vi "1.2.1-ParseYPR.vi"(9 "ASCII: VNYPR,":u8[](array[numeric])=[86, 78, 89, 80, 82, 44], 10 "Serial Byte":u8) -> (1 "Yaw":i16)   [LabVIEW 2010]
doc: "This VI parses Yaw, Pitch, and Roll (YPR) data from the VectorNav. In response to a YPR Read Request, the VectorNav will reply in the form \"$VNYPR,XX,-XXX.XX,-XXX.XX,+XXX.XX*XX\" (where X is a digit from 0-9). This string is in the form \"$<command type>,<access ID>, <yaw>,<pitch>,<roll>\".\n\nThe VI first waits for a $, then checks to make sure it has read \"VNYPR,\" correctly, then adds up each of the XX values and saves them appropriately. Since it receives these values one byte at a time , it must do some simple fixed point math to make sure the appropriate decimal value is saved."
uses:
  1.2.1-ParseYPR.ctl
panel:
  out "Heading (out)":T1 {"Yaw" format="%.19g"; "Pitch" format="%.19g"; "Roll" format="%.19g"}
  in  "Heading (in)":T1 {"Yaw" format="%.42g"; "Pitch" format="%.42g"; "Roll" format="%.42g"}
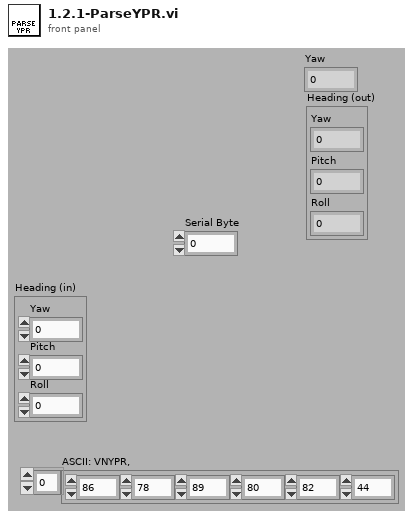
[diagram p1: front panel]
types:
  T1 = cluster{"Yaw":fxp<+/-,32,20>, "Pitch":fxp<+/-,32,20>, "Roll":fxp<+/-,32,20>}
  T2 = typedef "1.2.1-ParseYPR.ctl" = enum16{"Wait for $", "Check VNYPR", "Read numbers"}
  T3 = enum16{"Initialize", "Yaw", "Pitch", "Roll", "Done"}
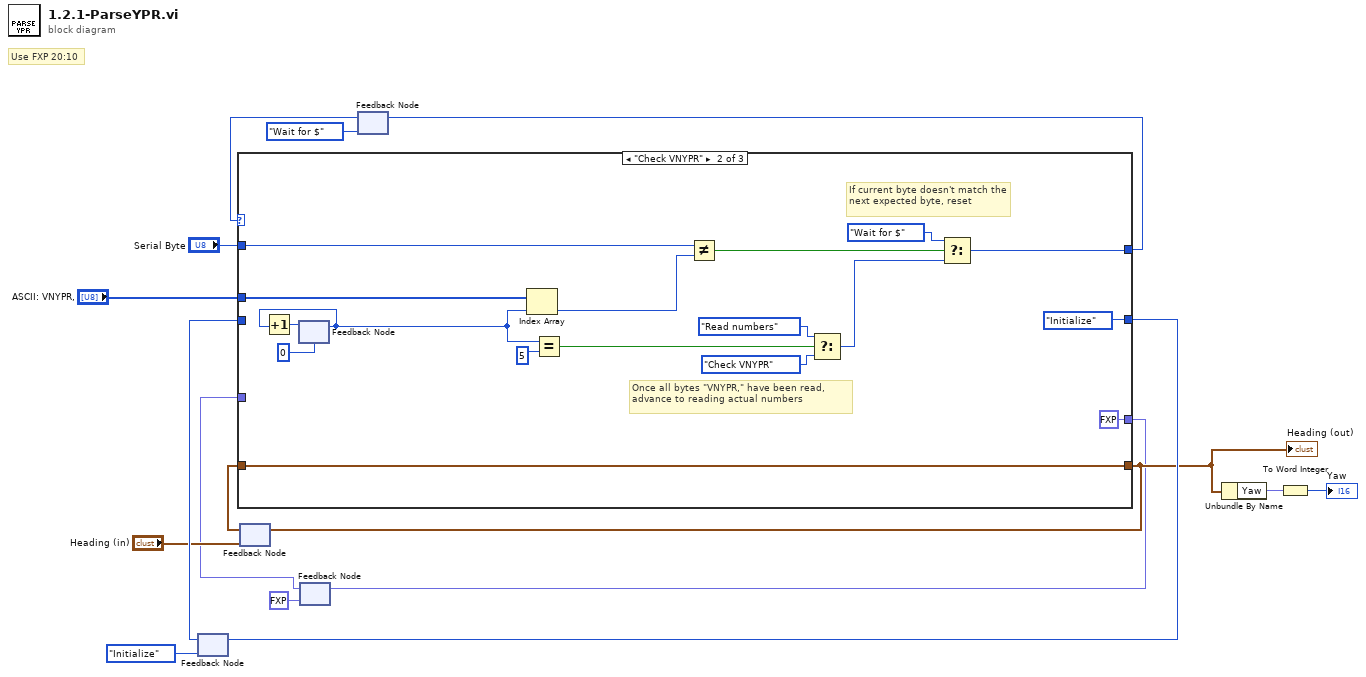
[diagram p0: block diagram]
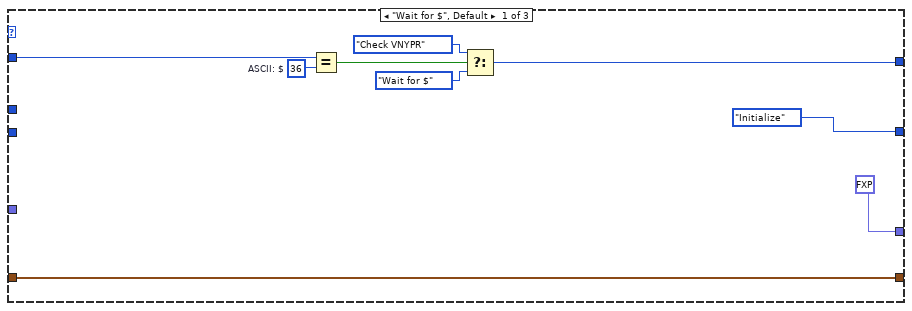
[diagram p2: hidden frame]
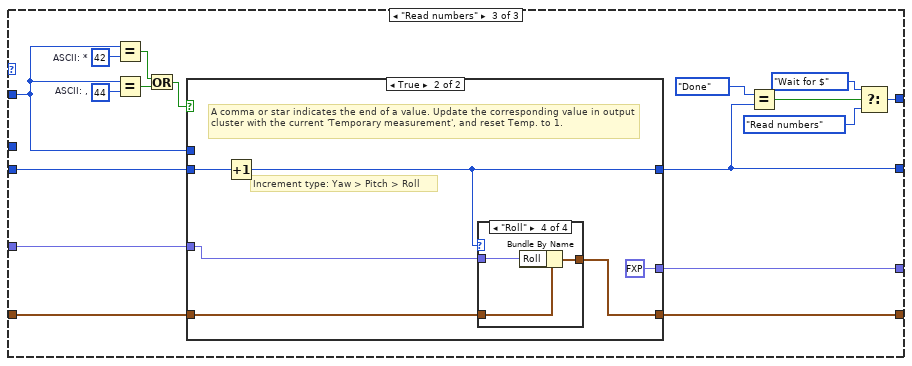
[diagram p3: hidden frame]
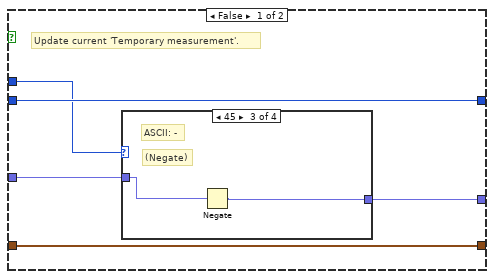
[diagram p4: hidden frame]
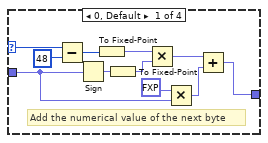
[diagram p5: hidden frame]
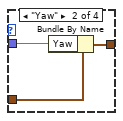
[diagram p9: hidden frame]
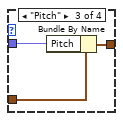
[diagram p10: hidden frame]
diagram:
  # "Use FXP 20:10"
  n1 = feedback #1(T3."Initialize" ("f")) -> (w11:T3)
  n2 = feedback #2("Heading (in)") -> (w5:T1)
  n3 = feedback #3(fxp<+/-,32,20> 1.0 ("Yaw")) -> (w3:fxp<+/-,32,20>)
  n4 = feedback #4(1.2.1-ParseYPR."Wait for $" ("1.3.1-ParseYPR")) -> (w14:T2)
  n5 = case shown="\"Check VNYPR\"" w14 {
    tunnel: [w22 w32 w47] -> w16
    tunnel: "Serial Byte" -> [w25 w39 w46]
    tunnel: [fxp<+/-,32,20> 1.0 ("Yaw") fxp<+/-,32,20> 1.0 ("Yaw") w48] -> w2
    tunnel: [w21 w40 w57] -> w4
    tunnel: w5 -> [w21 w40 w58]
    tunnel: [T3."Initialize" ("f") T3."Initialize" ("f") w55] -> w12
    tunnel: w11 -> [_ _ w56]
    tunnel: w3 -> [_ _ w43]
    tunnel: "ASCII: VNYPR," -> [_ w26 _]
    frame "Wait for $", Default {
      w24 = u8 36  # ASCII: $
      n6 = Equal?(x=w25, y=w24) -> (x = y?=w23:bool)
      n7 = Select(t=1.2.1-ParseYPR."Check VNYPR" ("1.3.1-ParseYPR"), s=w23, f=1.2.1-ParseYPR."Wait for $" ("1.3.1-ParseYPR")) -> (s? t:f=w22:T2)
    }
    frame "Check VNYPR" {
      # "If current byte doesn't match the next expected byte, reset"
      # "Once all bytes \"VNYPR,\" have been read, advance to reading actual numbers"
      n8 = feedback #5(0 ("Serial Byte")) -> (w27:i32)
      n9 = Increment(x=w27) -> (x+1=w28:i32)
      n10 = feedback-in #5(w28) -> ()
      n11 = Index Array(array=w26, index=w27) -> (element=w42:u8)
      n12 = Equal?(x=w27, y=5) -> (x = y?=w37:bool)
      n13 = Not Equal?(x=w39, y=w42) -> (x != y?=w41:bool)
      n14 = Select(t=1.2.1-ParseYPR."Read numbers" ("1.3.1-ParseYPR"), s=w37, f=1.2.1-ParseYPR."Check VNYPR" ("1.3.1-ParseYPR")) -> (s? t:f=w30:T2)
      n15 = Select(t=1.2.1-ParseYPR."Wait for $" ("1.3.1-ParseYPR"), s=w41, f=w30) -> (s? t:f=w32:T2)
    }
    frame "Read numbers" {
      w52 = u8 42  # ASCII: *
      w59 = u8 44  # ASCII: ,
      n16 = Equal?(x=w46, y=w52) -> (x = y?=w50:bool)
      n17 = Equal?(x=w46, y=w59) -> (x = y?=w51:bool)
      n18 = Or(x=w50, y=w51) -> (x .or. y?=w49:bool)
      n19 = case shown="True" w49 {
        tunnel: w58 -> [w64 w85]
        tunnel: [w64 w84] -> w57
        tunnel: [w63 w82] -> w55
        tunnel: w56 -> [w63 w83]
        tunnel: [w61 fxp<+/-,32,20> 1.0 ("Yaw")] -> w48
        tunnel: w46 -> [w62 _]
        tunnel: w43 -> [w60 w80]
        frame False {
          # "Update current 'Temporary measurement'."
          n20 = case shown="45" w62 {
            selector: w62 -> [w74 _ _ _]
            tunnel: [w72 w76 w77 w79] -> w61
            tunnel: w60 -> [w66 w76 w78 w79]
            frame 0, Default {
              # "Add the numerical value of the next byte"
              n21 = Subtract(x=w74, y=u8 48) -> (x-y=w70:u8)
              n22 = Sign(1:w66) -> (0:w69:fxp<+/-,2,2>)
              n23 = To Fixed-Point(number=w70) -> (fixed-point=w68:fxp<+/-,32,20>)  [unwired: 1 in]
              n24 = To Fixed-Point(number=w69) -> (fixed-point=w67:fxp<+/-,32,20>)  [unwired: 1 in]
              n25 = Multiply(x=w68, y=w67) -> (x*y=w65:fxp<+/-,32,20>)
              n26 = Multiply(x=fxp<+/-,20,10> 10.0 ("Yaw"), y=w66) -> (x*y=w75:fxp<+/-,52,30>)
              n27 = Add(x=w65, y=w75) -> (x+y=w72:fxp<+/-,32,20>)
            }
            frame 43 {
              # "ASCII: +"
            }
            frame 45 {
              # "(Negate)"
              # "ASCII: -"
              n28 = Negate(x=w78) -> (-x=w77:fxp<+/-,32,20>)
            }
            frame 46 {
              # "(Ignore decimal for now)"
              # "ASCII: ."
            }
          }
        }
        frame True {
          # "Increment type: Yaw > Pitch > Roll"
          # "A comma or star indicates the end of a value. Update the corresponding value in output cluster with the current 'Temporary measurement', and reset Temp. to 1."
          n29 = Increment(x=w83) -> (x+1=w82:T3)
          n30 = case shown="\"Roll\"" w82 {
            tunnel: [w86 w89 w92 w95] -> w84
            tunnel: w85 -> [w86 w88 w91 w94]
            tunnel: w80 -> [_ w87 w90 w93]
            frame "Initialize", Default {
            }
            frame "Yaw" {
              n31 = Bundle By Name(cluster=w88, "Yaw"=w87) -> (w89:T1)
            }
            frame "Pitch" {
              n32 = Bundle By Name(cluster=w91, "Pitch"=w90) -> (w92:T1)
            }
            frame "Roll" {
              n33 = Bundle By Name(cluster=w94, "Roll"=w93) -> (w95:T1)
            }
          }
        }
      }
      n34 = Equal?(x=T3."Done", y=w55) -> (x = y?=w53:bool)
      n35 = Select(t=1.2.1-ParseYPR."Wait for $" ("1.3.1-ParseYPR"), s=w53, f=1.2.1-ParseYPR."Read numbers" ("1.3.1-ParseYPR")) -> (s? t:f=w47:T2)
    }
  }
  "Heading (out)" <- w4
  n36 = feedback-in #1(w12) -> ()
  n37 = feedback-in #2(w4) -> ()
  n38 = feedback-in #3(w2) -> ()
  n39 = feedback-in #4(w16) -> ()
  n40 = Unbundle By Name(w4) -> ("Yaw"=w8:fxp<+/-,32,20>)
  n41 = To Word Integer(number=w8) -> (16bit integer=→"Yaw":i16)
